vi "Write Channel to Text Log File.vi"(6 "Data":dbl[](array[numeric]), 8 "error in (no error)":errorcluster, 9 "Channel Name in":string, 10 "Group Name in":string, 11 "Text Log File in":refnum<class "Text Log File.lvclass">) -> (0 "error out":errorcluster, 3 "Text Log File out":refnum<class "Text Log File.lvclass">)   [LabVIEW 2015, in "Waveform Data Logger Engine.lvlib" / "Text Log File.lvclass"]
doc: "Writes data to the text file using the specified delimiter and format string. The channel and group names are ignored. The header for the file should be written in advance using Write Log Header.vi."
uses:
  Text Log File.lvclass
  Text Log File.lvclass/Text Log File.ctl
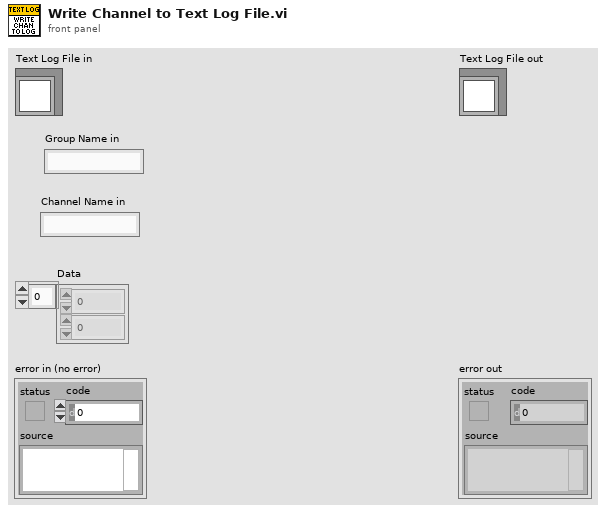
[diagram p1: front panel]
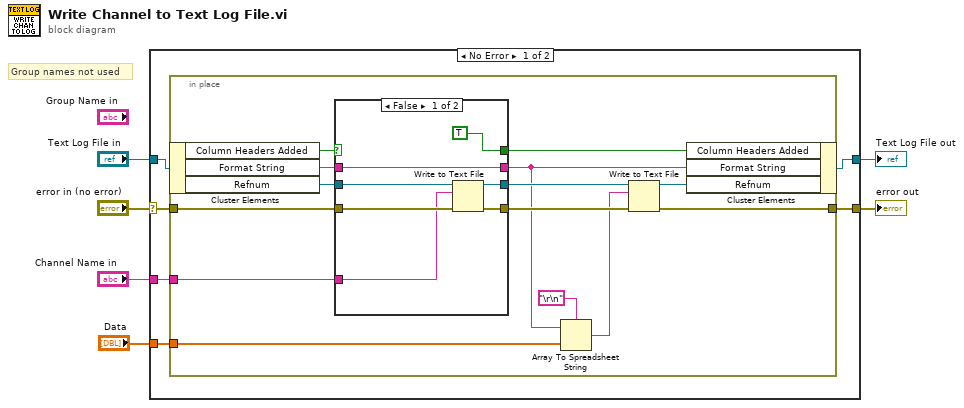
[diagram p0: block diagram]
diagram:
  # "Group names not used"
  n1 = case shown="No Error" "error in (no error)" {
    selector: "error in (no error)" -> [w8 w38]
    tunnel: [w12 w39] -> w6
    tunnel: "Data" -> [w11 _]
    tunnel: [w10 w38] -> w4
    tunnel: "Text Log File in" -> [w9 w39]
    tunnel: "Channel Name in" -> [w7 _]
    frame No Error {
      n2 = in-place {
        in-place-border: w8 -> [w21]
        in-place-border: w11 -> [w14]
        in-place-border: [w25] -> w10
        in-place-border: w7 -> [w22]
        n3 = in-place-cluster #1(w9) -> ("Column Headers Added"=w18:bool, "Format String"=w19:string, "Refnum"=w16:refnum<file>)
        n4 = case shown="False" w18 {
          selector: w18 -> [_ w37]
          tunnel: [w33 w35] -> w26
          tunnel: w16 -> [w32 w36]
          tunnel: [w31 w36] -> w23
          tunnel: [TRUE w37] -> w17
          tunnel: w22 -> [w27 _]
          tunnel: w21 -> [w30 w35]
          tunnel: [w28 w34] -> w20
          tunnel: w19 -> [w28 w34]
          frame False {
            n5 = Write to Text File(file (use dialog)=w32, text=w27, error in=w30) -> (refnum out=w31:refnum<file>, error out=w33:errorcluster)  [unwired: 1 in, 1 out]
          }
          frame True {
          }
        }
        n6 = Array To Spreadsheet String(delimiter (Tab)="\r\n", array=w14, 3:w20) -> (spreadsheet string=w24:string)
        n7 = Write to Text File(file (use dialog)=w23, text=w24, error in=w26) -> (refnum out=w15:refnum<file>, error out=w25:errorcluster)  [unwired: 1 in, 1 out]
        n8 = in-place-cluster #1("Column Headers Added"=w17, "Format String"=w20, "Refnum"=w15) -> (w12:refnum<class "Text Log File.lvclass">)
      }
    }
    frame Error {
    }
  }
  "error out" <- w4
  "Text Log File out" <- w6
